vi "Test_PublishUnnamed_PublicationIgnored_MediatorContinues.vi"(8 "error in (no error)":errorcluster, 11 "TestMediator In":refnum<class "TestMediationSemantics.lvclass">) -> (0 "error out":errorcluster, 3 "TestMediator Out":refnum<class "TestMediationSemantics.lvclass">)   [LabVIEW 2020, in "TestMediationSemantics.lvclass"]
uses:
  TestMediationSemantics.lvclass
  TestMediationSemantics.lvclass/TestMediationSemantics.ctl
  Source/Mediator/Mediator/Mediator.lvclass
  <vilib>/ActorFramework/Actor/Actor.lvclass
  Source/IMediator/IMediator Messages/Publish Msg/Publish Msg.lvclass
  <vilib>/ActorFramework/Stop Msg/Stop Msg.lvclass
  modules/composed-transport/Source/Concrete/QueueTransport/QueueTransport.lvclass
  Source/IMediator/IMediator Messages/Lock Publication Msg/Lock Publication Msg.lvclass
  Source/IMediator/IMediator/IMediator.lvclass
  593833ec-8834-4118-92b4-abe8c6b29c6b.vi
  modules/composed-event-logger/Source/Composed Log/LoggerReference/LoggerReference.lvclass
  modules/composed-event-logger/Source/String Control Sink/String Control Sink.lvclass
  C:/Git/mva-core/Source/IMediator/IMediator/IMediator.lvclass
  C:/Program Files (x86)/National Instruments/LabVIEW 2020/vi.lib/ActorFramework/Actor/Actor.lvclass
  C:/Git/mva-core/Source/Mediator/Mediator/Mediator.lvclass
  4b47616c-1ff1-4f07-a19a-833c042c696c.vi
  Source/IMediator/PublishRequest/PublishRequest.lvclass
  C:/Git/mva-core/modules/composed-transport/Source/ITransport/ITransport.lvclass
  C:/Git/mva-core/modules/composed-transport/Source/Concrete/QueueTransport/QueueTransport.lvclass
panel:
  out "Log":string
  out "Returned Error":errorcluster
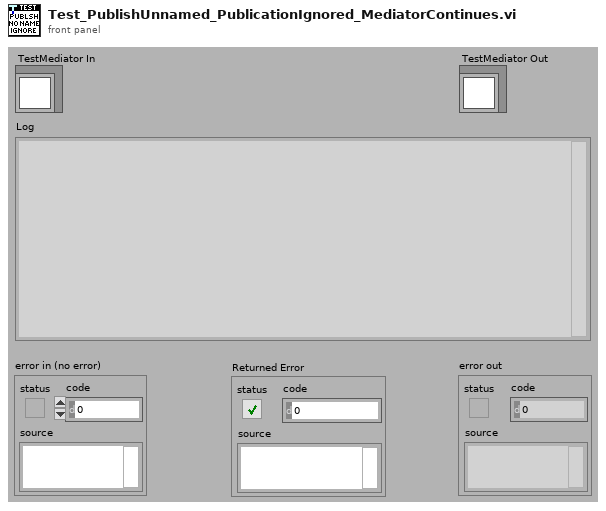
[diagram p1: front panel]
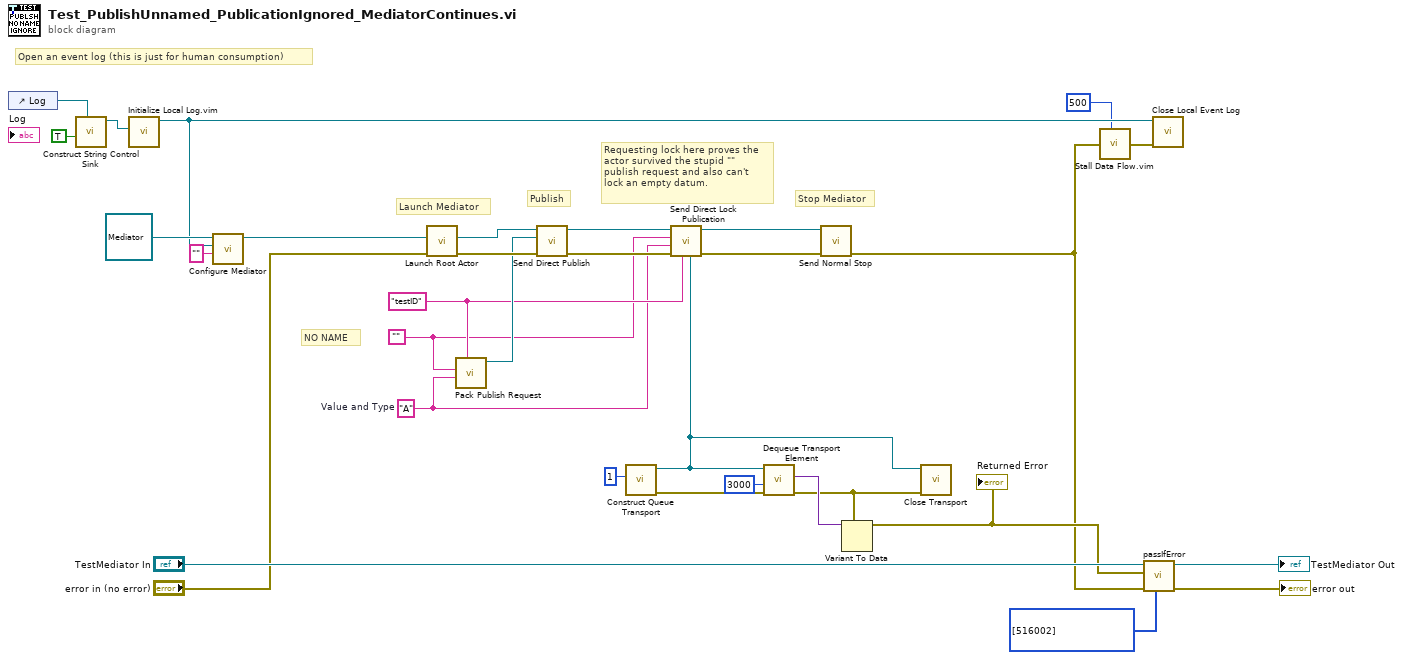
[diagram p0: block diagram]
diagram:
  w15 = "testID" ("Publisher ID")
  w13 = "" ("Datum Name")
  w14 = "A"  # Value and Type
  # "Open an event log (this is just for human consumption)"
  # "NO NAME"
  # "Launch Mediator"
  # "Stop Mediator"
  # "Requesting lock here proves the\nactor survived the stupid \"\"\npublish request and also can't\nlock an empty datum."
  # "Publish"
  n1 = control-ref of="Log"() -> (w8:refnum<vi>)
  n2 = call "Construct String Control Sink.vi"("Str Refnum"=w8, "AutoScroll?(F)"=TRUE) -> ("String Control Sink out"=w7:refnum<class "String Control Sink.lvclass">)  [unwired: 9 in]
  n3 = call "Initialize Local Log.vim"("Startup Sink(s)"=w7) -> ("Log Instance Reference"=w5:refnum<class "LoggerReference.lvclass">)  [unwired: 8 in, 2 out]
  n4 = call "Configure Mediator.vi"("Framework Instance Alias"="", "Event Log Instance"=w5, "Mediator in"=refnum<class "Mediator.lvclass"> refnum ("Mediator.lvlib:Mediator.lvclass")) -> ("Mediator out"=w27:refnum<class "Mediator.lvclass">)  [unwired: 8 in]
  n5 = call <vilib>:"Launch Root Actor.vi"("error in (no error)"="error in (no error)", "Actor"=w27) -> ("error out"=w22:errorcluster, "Actor's Enqueuer"=w26:refnum<class "Message Enqueuer.lvclass">)  [unwired: 8 in]
  n6 = call "Pack Publish Request.vi"("Publisher ID"=w15, "Value"=w14, "Datum Name"=w13) -> ("PublishRequest Out"=w21:refnum<class "PublishRequest.lvclass">)  [unwired: 7 in, 1 out]
  n7 = call "Send Direct Publish.vi"("error in (no error)"=w22, "PublishRequest"=w21, "Mediator Enqueuer"=w26) -> ("error out"=w18:errorcluster, "Mediator Enqueuer out"=w20:refnum<class "Message Enqueuer.lvclass">)  [unwired: 7 in]
  n8 = call "Construct Queue Transport.vi"("Max Queue Size (-1)"=1) -> ("error out"=w11:errorcluster, "QueueTransport"=w16:refnum<class "QueueTransport.lvclass">)  [unwired: 9 in]
  n9 = call "Send Direct Lock Publication.vi"("Return Error Transport"=w16, "Publisher ID"=w15, "error in (no error)"=w18, "Datum Type"=w14, "Datum Name"=w13, "Mediator Enqeuer"=w20) -> ("error out"=w17:errorcluster, "Mediator Enqueuer out"=w19:refnum<class "Message Enqueuer.lvclass">)  [unwired: 4 in]
  n10 = call "Dequeue Transport Element.vi"("error in (no error)"=w11, "Timeout In ms (-1)"=3000, "QueueTransport"=w16) -> ("error out"=w12:errorcluster, "Data"=w23:variant)  [unwired: 5 in, 2 out]
  n11 = call <vilib>:"Send Normal Stop.vi"("error in (no error)"=w17, "Message Enqueuer"=w19) -> ("error out"=w9:errorcluster)  [unwired: 9 in]
  n12 = Variant To Data(type=w12, Variant=w23) -> (data=w10:errorcluster)  [unwired: 1 in, 1 out]
  "Returned Error" <- w10
  n13 = call-dynamic "Close Transport.vi"("error in (no error)"=w12, "QueueTransport"=w16) -> ()  [unwired: 9 in, 1 out]
  n14 = call "Stall Data Flow.vim"("value in"=w9, "milliseconds to wait"=u32 500) -> ("value out"=w4:errorcluster)  [unwired: 1 out]
  n15 = call-dynamic "passIfError.vi"("passing error codes (default = any error code)"=i32[] [516002], "error in (no error)"=w9, "error"=w10, "TestCase in"="TestMediator In") -> ("error out"=→"error out":errorcluster, "TestCase out"=→"TestMediator Out":refnum<class "TestMediationSemantics.lvclass">)  [unwired: 6 in]
  n16 = call "Close Local Event Log.vi"("error in (no error)"=w4, "Log Instance"=w5) -> ()  [unwired: 9 in, 1 out]
